vi "Subvi SetLogFileName.vi"(1 "LogFileMax":u8, 2 "BaseAppPath":path, 3 "LogFileBaseName":string) -> (0 "LogFilePath":path)   [LabVIEW 2012]
panel:
  # "This Subvi sets up the filename for a rolling logfile.\nLogfiles are stored in a folder called Log under the\nBase App path. The log folder is created if it does\nnot exist\nInput:\n1. Logfile base name (string)\n2. Base App path (path)\n3. Max number of logfiles (U8)\nOutput:\n1. Logfile Path for this session (path)"
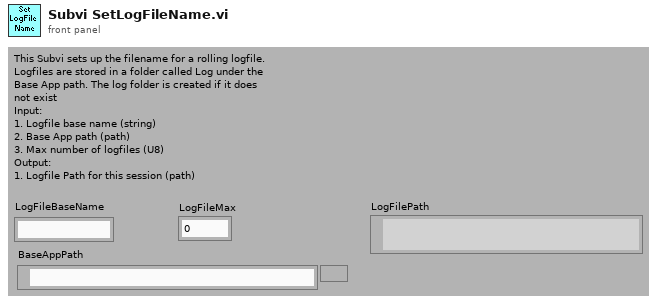
[diagram p1: front panel]
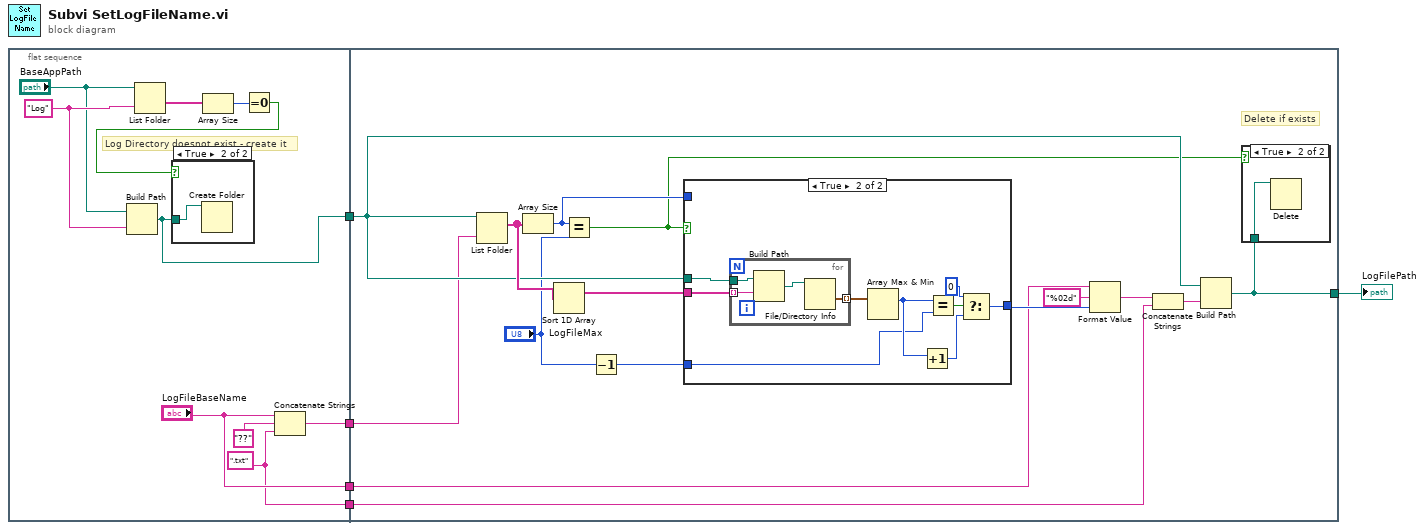
[diagram p0: block diagram]
diagram:
  n1 = flat-sequence {
    tunnel: [w9] -> w4
    tunnel: [w8] -> w3
    tunnel: ["LogFileBaseName"] -> w2
    tunnel: [w6] -> w1
    tunnel: [w17] -> w5
    tunnel: w4 -> [w24]
    tunnel: w3 -> [w23]
    tunnel: w2 -> [w22]
    tunnel: w1 -> [w21]
    frame #0 {
      w15 = "Log" ("pattern")
      w6 = ".txt" ("pattern")
      # "Log Directory doesnot exist - create it"
      n2 = Build Path(base path="BaseAppPath", name or relative path=w15) -> (appended path=w9:path)
      n3 = List Folder(path="BaseAppPath", pattern=w15) -> (folder names=w11:string[])  [unwired: 1 in, 4 out]
      n4 = Array Size(array=w11) -> (size(s)=w12:i32)
      n5 = Equal To 0?(x=w12) -> (x = 0?=w13:bool)
      n6 = case shown="True" w13 {
        tunnel: w9 -> [_ w16]
        frame False {
        }
        frame True {
          n7 = Create Folder(path (use dialog)=w16) -> ()  [unwired: 1 in, 4 out]
        }
      }
      n8 = Concatenate Strings("LogFileBaseName", "??" ("pattern"), w6) -> (w8:string)
    }
    frame #1 {
      # "Delete if exists"
      n9 = List Folder(path=w24, pattern=w23) -> (filenames=w31:string[])  [unwired: 1 in, 4 out]
      n10 = Array Size(array=w31) -> (size(s)=w29:i32)
      n11 = Sort 1D Array(array=w31) -> (sorted array=w30:string[])
      n12 = Equal?(x=w29, y="LogFileMax") -> (x = y?=w18:bool)
      n13 = Decrement(x="LogFileMax") -> (x-1=w19:u8)
      n14 = case shown="True" w18 {
        tunnel: w30 -> [_ w40]
        tunnel: w24 -> [_ w42]
        tunnel: w29 -> [w33 _]
        tunnel: [w33 w35] -> w27
        tunnel: w19 -> [_ w34]
        frame False {
        }
        frame True {
          n15 = for {
            tunnel: w40 -> [w46] mode=indexing
            tunnel: w42 -> [w45]
            tunnel: [w43] -> w41 mode=indexing
            n16 = Build Path(base path=w45, name or relative path=w46) -> (appended path=w44:path)
            n17 = File/Directory Info(path=w44) -> (last mod=w43:timestamp)  [unwired: 1 in, 6 out]
          }
          n18 = Array Max & Min(array=w41) -> (max index (indices)=w38:i32)  [unwired: 3 out]
          n19 = Increment(x=w38) -> (x+1=w37:i32)
          n20 = Equal?(x=w38, y=w34) -> (x = y?=w39:bool)
          n21 = Select(t=0 ("y"), s=w39, f=w37) -> (s? t:f=w35:i32)
        }
      }
      n22 = Format Value(string ("")=w22, format string="%02d", value (0)=w27) -> (output string=w28:string)
      n23 = Concatenate Strings(w28, w21) -> (w25:string)
      n24 = Build Path(base path=w24, name or relative path=w25) -> (appended path=w17:path)
      n25 = case shown="True" w18 {
        tunnel: w17 -> [_ w32]
        frame False {
        }
        frame True {
          n26 = Delete(path (use dialog)=w32) -> ()  [unwired: 1 in, 6 out]
        }
      }
    }
  }
  "LogFilePath" <- w5
